vi "例4.19 利用属性节点读取循环结构内外的数据.vi"() -> ()   [LabVIEW 2017]
panel:
  in  "停止":bool
  out "Y":dbl
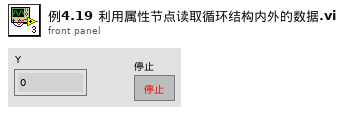
[diagram p1: front panel]
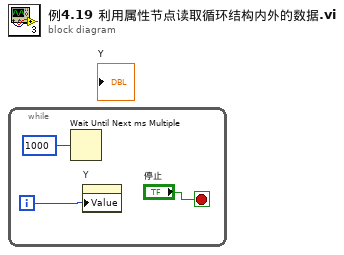
[diagram p0: block diagram]
diagram:
  n1 = while {
    i -> [w1]
    stop <- "停止" stop-if-true
    n2 = Wait Until Next ms Multiple(millisecond multiple=u32 1000 ("毫秒倍数")) -> ()  [unwired: 1 out]
    n3 = property on="Y" class="DigNum (严格)"("Value"=w1) -> ()  [unwired: 2 in, 2 out]
  }
